vi "Set_all_subsystem_buffers.vi"(5 "Group names":string[][](array[string]), 7 "Subsystem names":string[](array[string]), 8 "error in":errorcluster, 10 "Record rate (Hz)":dbl format="%#_13g", 11 "Refnum in":refnum<k34>) -> (0 "error out":errorcluster, 3 "Refnum out":refnum<k34>)   [LabVIEW 2017, in "labview-standard-library.lvlib"]
uses:
  labview-standard-library.lvlib
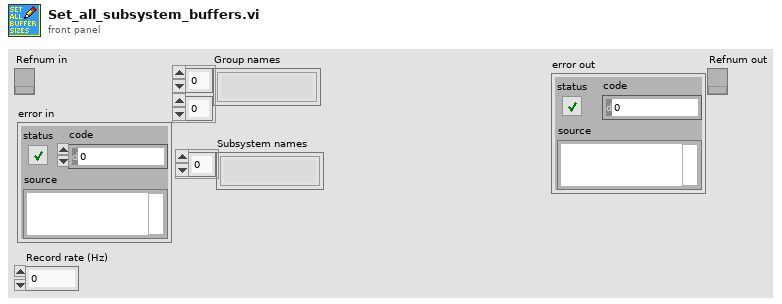
[diagram p1: front panel]
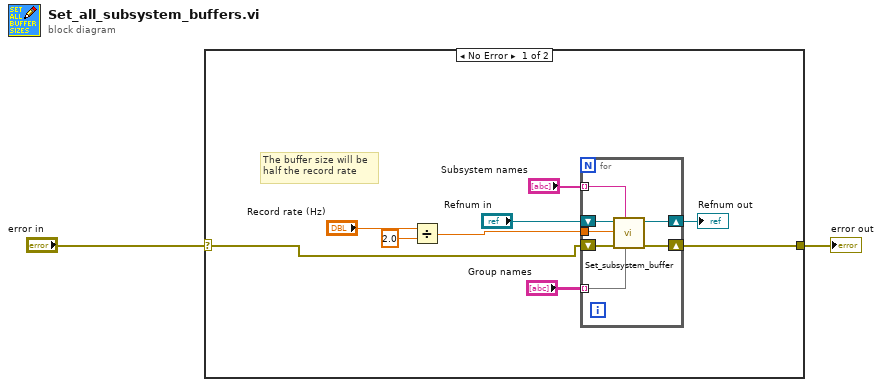
[diagram p0: block diagram]
diagram:
  n1 = case shown="No Error" "error in" {
    selector: "error in" -> [w3 w19]
    tunnel: [w9 w19] -> w2
    frame No Error {
      # "The buffer size will be\nhalf the record rate"
      n2 = Divide(x="Record rate (Hz)", y=2.0) -> (x/y=w6:dbl)
      n3 = for {
        tunnel: "Subsystem names" -> [w18] mode=indexing
        tunnel: "Group names" -> [w17] mode=indexing
        tunnel: w6 -> [w16]
        shift-right: [w15] -> w8
        shift-left: "Refnum in" -> [w14]
        shift-right: [w13] -> w9
        shift-left: w3 -> [w12]
        n4 = call "Set_subsystem_buffer.vi"("channel names"=w17, "Subsystem name in"=w18, "error in (no error)"=w12, "Buffer size"=w16, "Refnum in"=w14) -> ("error out"=w13:errorcluster, "Refnum out"=w15:refnum<k34>)  [unwired: 5 in]
      }
      "Refnum out" <- w8
    }
    frame Error {
    }
  }
  "error out" <- w2
